vi "Configure Digitize Current.vi"(0 "VISA resource name":refnum<visa-resource-name>, 5 "Manual Range":dbl=3.0 min=-3.0 max=3.0, 7 "Aperture Seconds":dbl=0.01616 min=8.333e-06 max=0.25 step=1e-06, 11 "error in (no error)":errorcluster) -> (4 "VISA resource name out":refnum<visa-resource-name>, 15 "error out":errorcluster)   [LabVIEW 2018, in "Keithley DMM7512.lvlib"]
doc: "This VI configures the Digitize Current and the related parameters."
uses:
  <instrlib>/Keithley DMM7512/Keithley DMM7512.lvlib
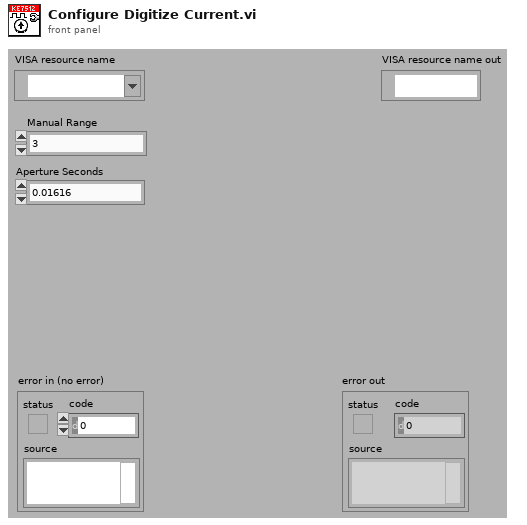
[diagram p1: front panel]
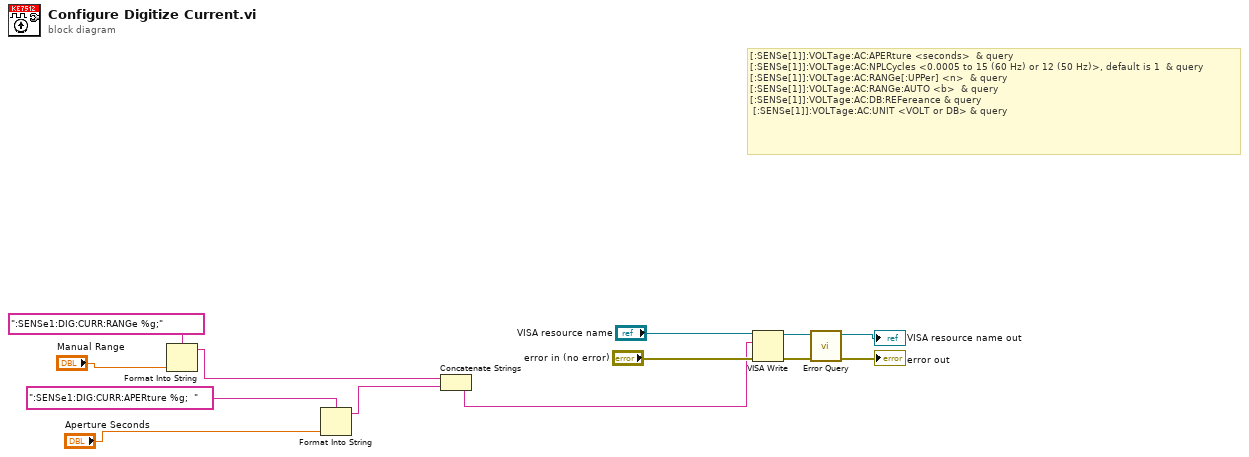
[diagram p0: block diagram]
diagram:
  # "[:SENSe[1]]:VOLTage:AC:APERture <seconds>  & query\n[:SENSe[1]]:VOLTage:AC:NPLCycles <0.0005 to 15 (60 Hz) or 12 (50 Hz)>, default is 1  & query\n[:SENSe[1]]:VOLTage:AC:RANGe[:UPPer] <n>  & query\n[:SENSe[1]]:VOLTage:AC:RANGe:AUTO <b>  & query\n[:SENSe[1]]:VOLTage:AC:DB:REFereance & query\n [:SENSe[1]]:VOLTage:AC:UNIT <VOLT or DB> & query"
  n1 = Format Into String(format string=":SENSe1:DIG:CURR:RANGe %g;", "Manual Range") -> (resulting string=w1:string)  [unwired: 2 in, 1 out]
  n2 = Format Into String(format string=":SENSe1:DIG:CURR:APERture %g;  ", "Aperture Seconds") -> (resulting string=w9:string)  [unwired: 2 in, 1 out]
  n3 = Concatenate Strings(w1, w9) -> (w8:string)
  n4 = VISA Write(VISA resource name="VISA resource name", write buffer=w8, error in (no error)="error in (no error)") -> (VISA resource name out=w7:refnum<visa-resource-name>, error out=w6:errorcluster)  [unwired: 1 out]
  n5 = call <instrlib>:"Error Query.vi"("error in (no error)"=w6, "VISA resource name"=w7) -> ("error out"=→"error out":errorcluster, "VISA resource name out"=→"VISA resource name out":refnum<visa-resource-name>)  [unwired: 6 in, 2 out]
